vi "overlap_calculator.vi"(0 "T1":dbl min=0.0, 2 "T2":dbl min=0.0, 3 "D":dbl min=0.0) -> (6 "overlap":dbl)   [LabVIEW 2015]
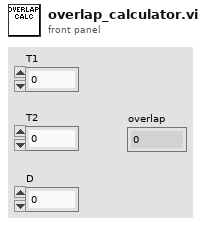
[diagram p1: front panel]
types:
  T1 = enum16{"D<=T1-T2 ^ D<T1", "D<T1 ^ D>T1-T2", "D>=T1"}
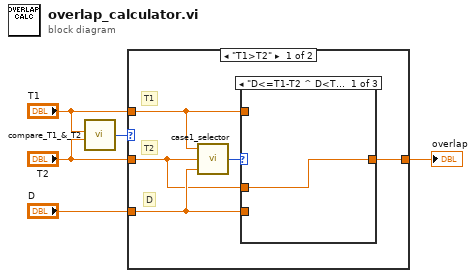
[diagram p0: block diagram]
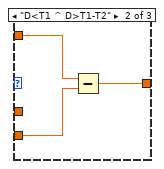
[diagram p2: hidden frame]
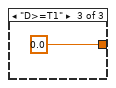
[diagram p3: hidden frame]
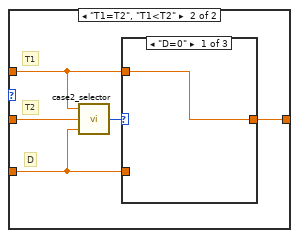
[diagram p4: hidden frame]
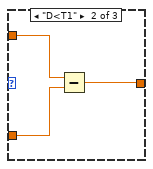
[diagram p5: hidden frame]
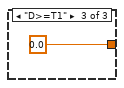
[diagram p6: hidden frame]
diagram:
  n1 = call "compare_T1_&_T2.vi"("T1"="T1", "T2"="T2") -> ("Result"=w1:enum16{"T1>T2", "T1=T2", "T1<T2"})  [unwired: 6 in]
  n2 = case shown="\"T1>T2\"" w1 {
    tunnel: "T1" -> [w8 w18]
    tunnel: "T2" -> [w6 w20]
    tunnel: "D" -> [w7 w16]
    tunnel: [w9 w17] -> w5
    frame "T1>T2" {
      # "D"
      # "T2"
      # "T1"
      n3 = call "case1_selector.vi"("T1"=w8, "T2"=w6, "Delay"=w7) -> ("overlap select"=w10:T1)  [unwired: 4 in]
      n4 = case shown="\"D<=T1-T2 ^ D<T1\"" w10 {
        tunnel: w8 -> [_ w14 _]
        tunnel: [w11 w12 0.0] -> w9
        tunnel: w7 -> [_ w13 _]
        tunnel: w6 -> [w11 _ _]
        frame "D<=T1-T2 ^ D<T1" {
        }
        frame "D<T1 ^ D>T1-T2" {
          n5 = Subtract(x=w14, y=w13) -> (x-y=w12:dbl)
        }
        frame "D>=T1" {
        }
      }
    }
    frame "T1=T2", "T1<T2" {
      # "D"
      # "T2"
      # "T1"
      n6 = call "case2_selector.vi"("T1"=w18, "T2"=w20, "Delay"=w16) -> ("Case 2 selector"=w19:enum16{"D=0", "D<T1", "D>=T1"})  [unwired: 4 in]
      n7 = case shown="\"D=0\"" w19 {
        tunnel: w18 -> [w21 w23 _]
        tunnel: [w21 w24 0.0] -> w17
        tunnel: w16 -> [_ w22 _]
        frame "D=0" {
        }
        frame "D<T1" {
          n8 = Subtract(x=w23, y=w22) -> (x-y=w24:dbl)
        }
        frame "D>=T1" {
        }
      }
    }
  }
  "overlap" <- w5
